vi "Open Item.vi"(8 "error in (no error)":errorcluster, 10 "Item name":string, 11 "Measure Object in":refnum<class "Measure Object.lvclass">) -> (0 "error out":errorcluster, 3 "Measure Object out":refnum<class "Measure Object.lvclass">)   [LabVIEW 2015, in "Measure Object.lvclass"]
uses:
  Measure Object.lvclass
  <vilib>/ActorFramework/Actor/Actor.lvclass/Actor.ctl
  Measure Object Messages/Open Item Msg/Open Item Msg.lvclass/Open Item Msg.ctl
  <vilib>/ActorFramework/Message Enqueuer/Message Enqueuer.lvclass/Message Enqueuer.ctl
  <vilib>/ActorFramework/Message Enqueuer/Enqueue.vi
  <vilib>/ActorFramework/Message Priority Queue/Priority Enqueue.vi
  Measure Object Messages/Open Item Msg/Open Item Msg.lvclass
  Measure Object Messages/Open Front Panel Msg/Open Front Panel Msg.lvclass
  <vilib>/ActorFramework/Actor/Actor.lvclass
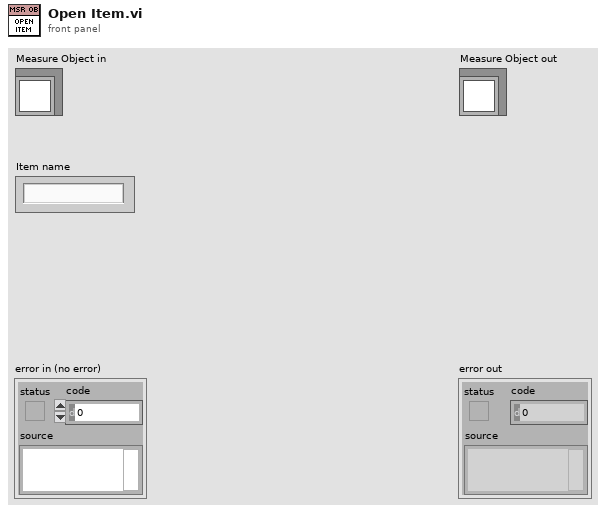
[diagram p1: front panel]
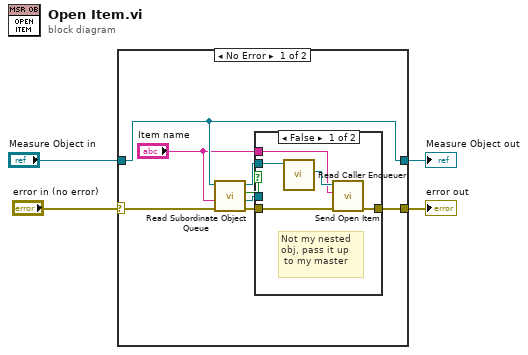
[diagram p0: block diagram]
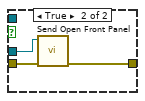
[diagram p2: hidden frame]
diagram:
  n1 = case shown="No Error" "error in (no error)" {
    selector: "error in (no error)" -> [w8 w22]
    tunnel: [w5 w22] -> w3
    tunnel: [w12 w21] -> w1
    tunnel: "Measure Object in" -> [w12 w21]
    frame No Error {
      n2 = call-dynamic "Read Subordinate Object Queue.vi"("error in (no error)"=w8, "Name"="Item name", "Measure Object in"=w12) -> ("error out"=w6:errorcluster, "Object Enqueuer"=w9:refnum<class "Message Enqueuer.lvclass">, "Found?"=w11:bool, "Measure Object out"=w10:refnum<class "Measure Object.lvclass">)  [unwired: 5 in]
      n3 = case shown="False" w11 {
        tunnel: w10 -> [w17 _]
        tunnel: w9 -> [_ w20]
        tunnel: "Item name" -> [w15 _]
        tunnel: w6 -> [w14 w19]
        tunnel: [w13 w18] -> w5
        frame False {
          # "Not my nested \nobj, pass it up\n to my master"
          n4 = call <vilib>:"Read Caller Enqueuer.vi"("Actor"=w17) -> ("Caller Enqueuer"=w16:refnum<class "Message Enqueuer.lvclass">)  [unwired: 10 in]
          n5 = call "Send Open Item.vi"("error in (no error)"=w14, "Item name"=w15, "Message Enqueuer"=w16) -> ("error out"=w13:errorcluster)  [unwired: 7 in, 1 out]
        }
        frame True {
          n6 = call "Send Open Front Panel.vi"("error in (no error)"=w19, "Message Enqueuer"=w20) -> ("error out"=w18:errorcluster)  [unwired: 8 in, 1 out]
        }
      }
    }
    frame Error {
    }
  }
  "error out" <- w3
  "Measure Object out" <- w1
